vi "Open.vi"(4 "Gyro Full Scale Range":T2, 6 "Accel Full Scale Range":T3, 7 "I2C Channel":u8, 8 "Error In":errorcluster, 9 "Clock Source":T1, 10 "I2C Slave Address":T10=enum."0x69", 11 "LINX Resource":T4) -> (0 "Error Out":errorcluster, 3 "LINX Resource":T4)   [LabVIEW 2019, in "LMH-LINX.lvlib" / "MPU60X0.lvlib"]
doc: "Initializes the MPU-60X0 device setting the clock source and the full ranges for the accelerometer and gyro.\n\nOriginal Code Contributed By NathanB"
uses:
  <vilib>/MakerHub/LINX/Public/Sensors/Accelerometer/MPU60X0/MPU60X0.lvlib
  <vilib>/MakerHub/LINX/Public/Sensors/Accelerometer/MPU60X0/DeviceAddresses.ctl
  <vilib>/MakerHub/LINX/Private/Type Defs/LINX Ref.ctl
  <vilib>/MakerHub/LINX/Private/Type Defs/Platform.ctl
  <vilib>/MakerHub/LINX/Private/Type Defs/Interface.ctl
  <vilib>/MakerHub/LINX/Private/Device/Type Defs/LINX Device Config.ctl
  <vilib>/MakerHub/LINX/Private/Device/Type Defs/TCP Config.ctl
  <vilib>/MakerHub/LINX/Private/Device/Type Defs/Channels.ctl
  <vilib>/MakerHub/LINX/Public/Sensors/Accelerometer/MPU60X0/AccelFullScaleRanges.ctl
  <vilib>/MakerHub/LINX/Public/Sensors/Accelerometer/MPU60X0/GyroFullScaleRanges.ctl
  <vilib>/MakerHub/LINX/Public/Sensors/Accelerometer/MPU60X0/Clock Source.ctl
  <vilib>/MakerHub/LINX/LMH-LINX.lvlib
  <vilib>/MakerHub/LINX/Private/Device/Device.lvlib
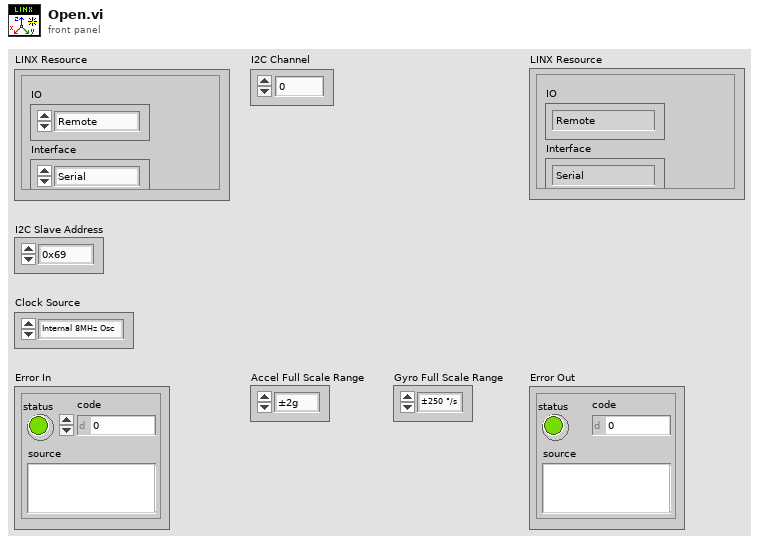
[diagram p1: front panel]
types:
  T1 = typedef "LMH-LINX.lvlib/MPU60X0.lvlib/Clock Source.ctl" = enum8{"Internal 8MHz Osc", "PLL with X Gyro Ref", "PLL with Y Gyro Ref", "PLL with Z Gyro Ref", "PLL with ext 32.768 KHz Ref", "PLL with ext 19.2 MHz Ref", "Reserved", "Hold in reset"}
  T2 = typedef "LMH-LINX.lvlib/MPU60X0.lvlib/GyroFullScaleRanges.ctl" = enum8{"±250 °/s", "±500 °/s", "±1000 °/s", "±2000 °/s"}
  T3 = typedef "LMH-LINX.lvlib/MPU60X0.lvlib/AccelFullScaleRanges.ctl" = enum16{"±2g", "±4g", "±8g", "±16g"}
  T4 = typedef "LMH-LINX.lvlib/LINX Ref.ctl" = cluster{"IO":T5, "Interface":T6, "LINX Device Config":T7}
  T5 = typedef "LMH-LINX.lvlib/Platform.ctl" = enum16{"Remote", "Local"}
  T6 = typedef "LMH-LINX.lvlib/Interface.ctl" = enum16{"Serial", "TCP"}
  T7 = typedef "LMH-LINX.lvlib/Device.lvlib/LINX Device Config.ctl" = cluster{"Interface":T6, "COM Port":refnum<visa-resource-name>, "TCP Configuration":T8, "Device Family":u8, "Device ID":u8, "Device Name":string, "TCP Ref":refnum<k5>, "Channels":T9}
  T8 = typedef "LMH-LINX.lvlib/Device.lvlib/TCP Config.ctl" = cluster{"IP Address":string, "Port":u16}
  T9 = typedef "LMH-LINX.lvlib/Channels.ctl" = cluster{"DI":u8[], "DO":u8[], "AI":u8[], "AO":u8[], "PWM":u8[], "QE":u8[], "UART":u8[], "I2C 2":u8[], "SPI":u8[], "CAN":u8[], "Servo":u8[], "AI Ref (V)":dbl, "AI Resolution (Bits)":u8, "AO Ref (V)":dbl, "AO Resolution (Bits)":u8}
  T10 = typedef "LMH-LINX.lvlib/MPU60X0.lvlib/DeviceAddresses.ctl" = enum16{"0x68", "0x69"}
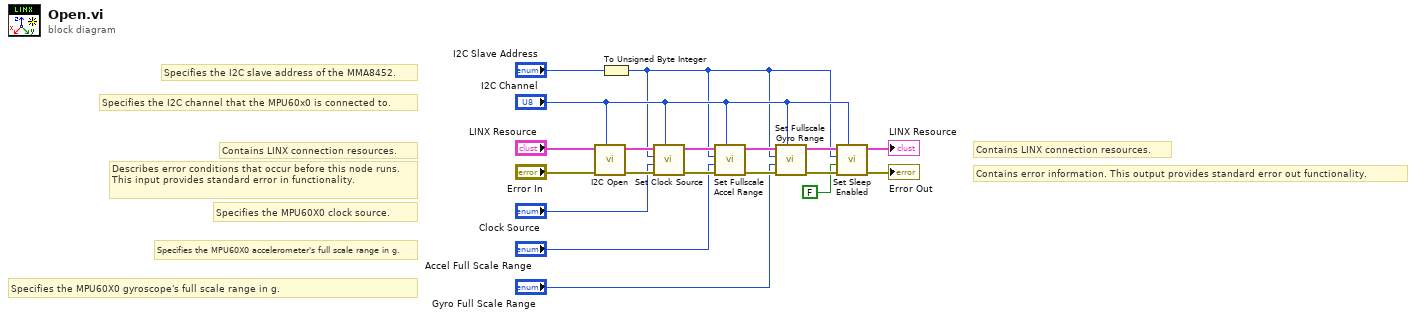
[diagram p0: block diagram]
diagram:
  # "Specifies the MPU60X0 gyroscope's full scale range in g."
  # "Specifies the MPU60X0 accelerometer's full scale range in g."
  # "Specifies the MPU60X0 clock source."
  # "Specifies the I2C slave address of the MMA8452."
  # "Specifies the I2C channel that the MPU60x0 is connected to."
  # "Contains LINX connection resources."
  # "Describes error conditions that occur before this node runs. This input provides standard error in functionality."
  # "Contains LINX connection resources."
  # "Contains error information. This output provides standard error out functionality."
  n1 = call <vilib>:"I2C Open.vi"("I2C Channel (0)"="I2C Channel", "Error In"="Error In", "LINX Resource"="LINX Resource") -> ("Error Out"=w7:errorcluster, "LINX Resource"=w9:T4)  [unwired: 7 in]
  n2 = To Unsigned Byte Integer(number="I2C Slave Address") -> (unsigned 8bit integer=w5:u8)
  n3 = call <vilib>:"Set Clock Source.vi"("I2C Channel"="I2C Channel", "Error In"=w7, "Clock Source"="Clock Source", "Device Address"=w5, "LINX Resource"=w9) -> ("Error Out"=w18:errorcluster, "LINX Resource"=w13:T4)  [unwired: 5 in]
  n4 = call <vilib>:"Set Fullscale Accel Range.vi"("I2C Channel"="I2C Channel", "Error In"=w18, "Accel Full Scale Range"="Accel Full Scale Range", "Device Address"=w5, "LINX Resource"=w13) -> ("Error Out"=w17:errorcluster, "LINX Resource"=w12:T4)  [unwired: 5 in]
  n5 = call <vilib>:"Set Fullscale Gyro Range.vi"("I2C Channel"="I2C Channel", "Error In"=w17, "Gyro Full Scale Range"="Gyro Full Scale Range", "Device Address"=w5, "LINX Resource"=w12) -> ("Error Out"=w16:errorcluster, "LINX Resource"=w19:T4)  [unwired: 5 in]
  n6 = call <vilib>:"Set Sleep Enabled.vi"("I2C Channel"="I2C Channel", "Error In"=w16, "Sleep?"=FALSE, "Device Address"=w5, "LINX Resource"=w19) -> ("Error Out"=→"Error Out":errorcluster, "LINX Resource"=→"LINX Resource":T4)  [unwired: 5 in]
